vi "rad_Modify and Deploy RT-INI.vi"(5 "password":string, 6 "Timeout msec (30s)":u32=30000, 7 "user (admin)":string="admin", 8 "error in (no error)":errorcluster, 9 "Run at Startup?":bool, 10 "Target settings":T1={"Hostname"="", "Serial number"="", "Product name"="", "Product code"=0, "System status"="", "Credential type"=enum."None/Unlocked", "User added?"=FALSE, "Primary NIC"={"MAC address"="", "IP Address Request Mode"=2, "IP address"="", "Subnet mask"="", "Gateway"="", "DNS server"=""}} {"Primary NIC"."IP Address Request Mode" items=["Static"=1, "DHCP/Link-Local"=2, "Link-Local Only"=4, "DHCP Only"=8]}, 11 "temp folder":path) -> (0 "error out":errorcluster)   [LabVIEW 2013]
uses:
  Targets/TypeDefs/rad_Target Information.ctl
  Targets/TypeDefs/rad_Target Network Settings.ctl
  <vilib>/Utility/config.llb/Write Key (Boolean).vi
  <vilib>/nisyscfg/Save Changes (Hardware).vi
  <vilib>/nisyscfg/Close (Hardware).vi
  <vilib>/nisyscfg/Close (System).vi
  <vilib>/Utility/config.llb/NI_LVConfig.lvlib
  <resource>/objmgr/nisysapi.rc
  <vilib>/nisyscfg/nisyscfg.lvlib
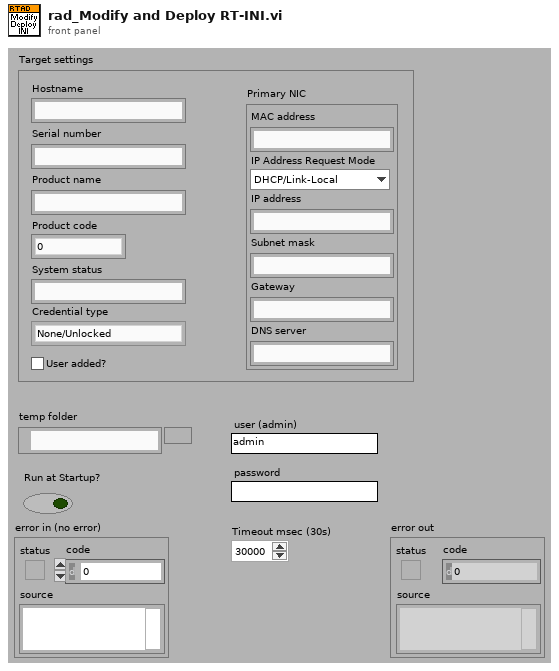
[diagram p1: front panel]
types:
  T1 = typedef "rad_Target Information.ctl" = cluster{"Hostname":string, "Serial number":string, "Product name":string, "Product code":i32, "System status":string, "Credential type":enum16{"None/Unlocked", "FTP Password", "NIAuth Credentials"}, "User added?":bool, "Primary NIC":T2}
  T2 = typedef "rad_Target Network Settings.ctl" = cluster{"MAC address":string, "IP Address Request Mode":i32, "IP address":string, "Subnet mask":string, "Gateway":string, "DNS server":string}
  T3 = enum16{"None/Unlocked", "FTP Password", "NIAuth Credentials"}
  T4 = typedef "NI_LVConfig.lvlib/Config Data RefNum.ctl" = refnum<k1>
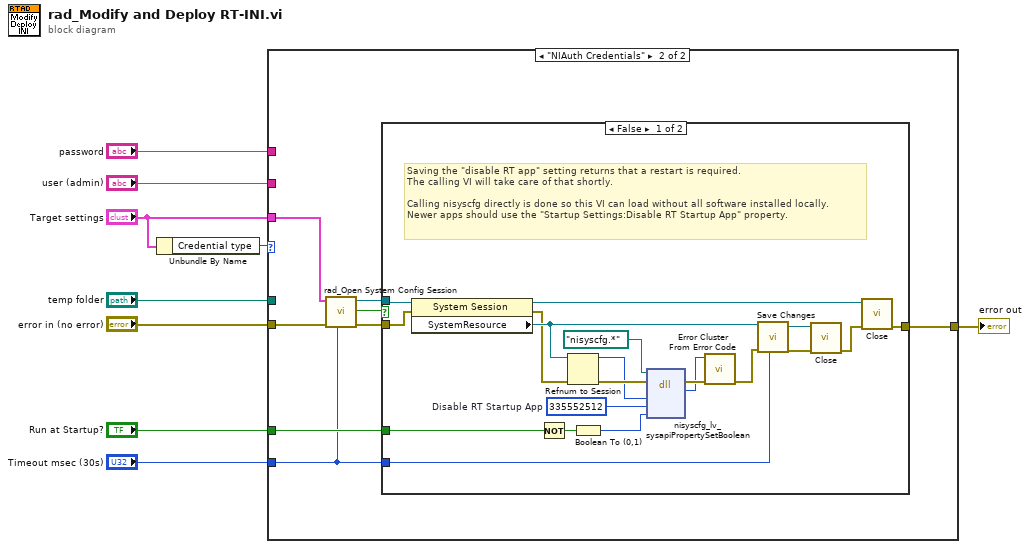
[diagram p0: block diagram]
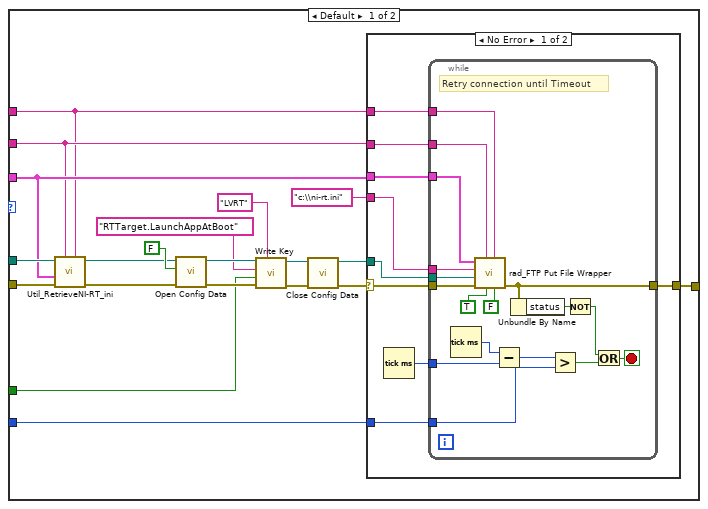
[diagram p2: hidden frame]
diagram:
  n1 = Unbundle By Name("Target settings") -> ("Credential type"=w1:T3)
  n2 = case shown="\"NIAuth Credentials\"" w1 {
    tunnel: "Run at Startup?" -> [w24 w58]
    tunnel: "Timeout msec (30s)" -> [w21 w57]
    tunnel: "user (admin)" -> [w11 _]
    tunnel: "password" -> [w10 _]
    tunnel: [w17 w59] -> w5
    tunnel: "temp folder" -> [w16 _]
    tunnel: "error in (no error)" -> [w14 w63]
    tunnel: "Target settings" -> [w12 w64]
    frame Default {
      n3 = call "Util_RetrieveNI-RT_ini.vi"("password"=w10, "user (admin)"=w11, "error in"=w14, "Target settings"=w12, "temp folder"=w16) -> ("error out"=w13:errorcluster, "Ini File Path"=w15:path)  [unwired: 5 in]
      n4 = call <vilib>:"Open Config Data.vi"("error in (no error)"=w13, "create file if necessary (T)"=FALSE, "configuration file path"=w15) -> ("error out"=w28:errorcluster, "refnum"=w27:T4)  [unwired: 6 in, 1 out]
      n5 = call-poly <vilib>:"Write Key.vi"("section"="LVRT", "error in (no error)"=w28, "value"=w24, "key"="RTTarget.LaunchAppAtBoot", "refnum"=w27) -> ("error out"=w22:errorcluster, "refnum out"=w23:T4)  [unwired: 4 in, 1 out]
      n6 = call <vilib>:"Close Config Data.vi"("error in (no error)"=w22, "refnum"=w23) -> ("error out"=w20:errorcluster, "file path"=w18:path)  [unwired: 8 in]
      n7 = case shown="No Error" w20 {
        selector: w20 -> [w37 w56]
        tunnel: [w36 w56] -> w17
        tunnel: w21 -> [w35 _]
        tunnel: "c:\\ni-rt.ini" ("remote path") -> [w34 _]
        tunnel: w18 -> [w33 _]
        tunnel: w12 -> [w32 _]
        tunnel: w11 -> [w31 _]
        tunnel: w10 -> [w30 _]
        frame No Error {
          n8 = Tick Count (ms)() -> (millisecond timer value=w38:u32)
          n9 = while {
            tunnel: w37 -> [w48]
            tunnel: w38 -> [w54]
            tunnel: [w47] -> w36
            tunnel: w35 -> [w46]
            tunnel: w34 -> [w45]
            tunnel: w33 -> [w44]
            tunnel: w32 -> [w43]
            tunnel: w31 -> [w42]
            tunnel: w30 -> [w41]
            stop <- w50 stop-if-true
            # "Retry connection until Timeout"
            n10 = Tick Count (ms)() -> (millisecond timer value=w55:u32)
            n11 = call "rad_FTP Put File Wrapper.vi"("active (F)"=FALSE ("active (T)"), "password"=w41, "binary (T)"=TRUE ("binary (F)"), "user (admin)"=w42, "error in (no error)"=w48, "local path"=w44, "remote path"=w45, "Target settings"=w43) -> ("error out"=w47:errorcluster)  [unwired: 3 in]
            n12 = Subtract(x=w55, y=w54) -> (x-y=w53:u32)
            n13 = Unbundle By Name(w47) -> ("status"=w49:bool)
            n14 = Greater?(x=w53, y=w46) -> (0:w51:bool)
            n15 = Not(x=w49) -> (.not. x?=w52:bool)
            n16 = Or(x=w52, y=w51) -> (x .or. y?=w50:bool)
          }
        }
        frame Error {
        }
      }
    }
    frame "NIAuth Credentials" {
      n17 = call "rad_Open System Config Session.vi"("Timeout ms (4000)"=w57, "error in (no error)"=w63, "Target settings"=w64) -> ("error out"=w60:errorcluster, "Cancelled"=w62:bool, "Session out"=w61:refnum<k21>)  [unwired: 5 in, 1 out]
      n18 = case shown="False" w62 {
        tunnel: w61 -> [w84 _]
        tunnel: w60 -> [w83 w85]
        tunnel: [w77 w85] -> w59
        tunnel: w58 -> [w82 _]
        tunnel: w57 -> [w76 _]
        frame False {
          w71 = u32 335552512  # Disable RT Startup App
          # "Saving the \"disable RT app\" setting returns that a restart is required.\nThe calling VI will take care of that shortly.\n\nCalling nisyscfg directly is done so this VI can load without all software installed locally.\nNewer apps should use the \"Startup Settings:Disable RT Startup App\" property."
          n19 = property class="System Session"(reference=w84, error in=w83) -> (reference out=w81:refnum<k21>, error out=w68:errorcluster, "SystemResource"=w69:refnum<k20>)
          n20 = Not(x=w82) -> (.not. x?=w66:bool)
          n21 = Refnum to Session(4:w68, 7:w69) -> (0:w75:errorcluster, 3:w70:u64)
          n22 = Boolean To (0,1)(Boolean=w66) -> (0, 1=w65:i16)
          n23 = dll-call lib="nisyscfg.dll" fn="nisyscfg_lv_sysapiPropertySetBoolean"(path in=path "nisyscfg.*", error in=w75, "resource"=w70, "attribute"=w71, "value"=w65) -> (error out=w74:errorcluster, "status"=w72:i32)  [unwired: 4 in, 1 out]
          n24 = call <vilib>:"Error Cluster From Error Code.vi"("error in (no error)"=w74, "error code (0)"=w72) -> ("error out"=w67:errorcluster)  [unwired: 2 in, 5 out]
          n25 = call-poly <vilib>:"Save Changes.vi"("Remote Timeout (300,000 ms)"=w76, "error in (no error)"=w67, "Resource in"=w69) -> ("error out"=w79:errorcluster, "Resource out"=w80:refnum<k20>)  [unwired: 5 in, 2 out]
          n26 = call-poly <vilib>:"Close.vi"("error in (no error)"=w79, "Resource in"=w80) -> ("error out"=w78:errorcluster)  [unwired: 9 in]
          n27 = call-poly <vilib>:"Close.vi"("error in (no error)"=w78, "Session in"=w81) -> ("error out"=w77:errorcluster)  [unwired: 9 in]
        }
        frame True {
        }
      }
    }
  }
  "error out" <- w5
